vi "DeadbandJoystick.vi"(11 "InputArray":dbl[](array[numeric])) -> (3 "OutputArray":dbl[](array[numeric]))   [LabVIEW 2019]
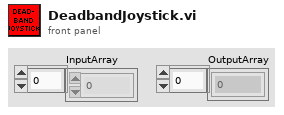
[diagram p1: front panel]
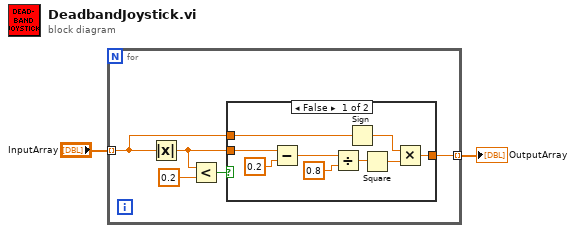
[diagram p0: block diagram]
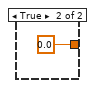
[diagram p2: hidden frame]
diagram:
  n1 = for {
    tunnel: "InputArray" -> [w4] mode=indexing
    tunnel: [w3] -> w1 mode=indexing
    n2 = Absolute Value(x=w4) -> (abs(x)=w5:dbl)
    n3 = Less?(x=w5, y=0.2) -> (x < y?=w7:bool)
    n4 = case shown="False" w7 {
      tunnel: w5 -> [w16 _]
      tunnel: [w8 0.0] -> w3
      tunnel: w4 -> [w11 _]
      frame False {
        n5 = Subtract(x=w16, y=0.2) -> (x-y=w14:dbl)
        n6 = Divide(x=w14, y=0.8) -> (x/y=w12:dbl)
        n7 = Sign(1:w11) -> (0:w9:dbl)
        n8 = Square(x=w12) -> (x^2=w10:dbl)
        n9 = Multiply(x=w9, y=w10) -> (x*y=w8:dbl)
      }
      frame True {
      }
    }
  }
  "OutputArray" <- w1
